vi "AB_Engine_Check_for_nonVI_Link.vi"(1 "buttons":u16, 2 "type":T1) -> (7 "nonVIlink":bool)   [LabVIEW 2020]
uses:
  <vilib>/Utility/lvfile.llb/LVFileType.ctl
  <vilib>/Utility/lvfile.llb/NI_FileType.lvlib
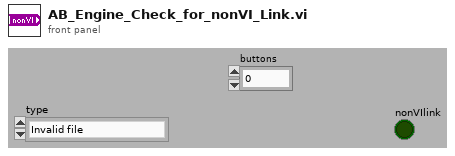
[diagram p1: front panel]
types:
  T1 = typedef "NI_FileType.lvlib/LVFileType.ctl" = enum32{"Invalid file", "Unknown type", "Instrument", "Control", "Polymorphic VI", "Project", "Library", "LVClass", "XControl", "XNode", "Shared library", ".NET assembly", "ActiveX interface", "CIN", "Run-time menu", "Palette menu", "Help file", "LLB", "XNode Edit Dependency", "Class Private Data Control", "Statechart", "MathScript .m file", "Ladder Diagram", "LVLibp", "XNode Build Dependency"}
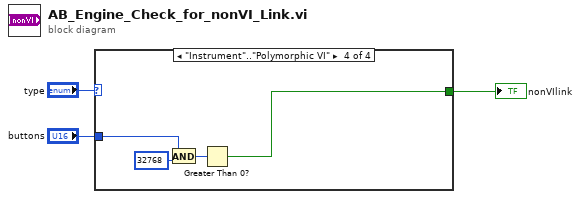
[diagram p0: block diagram]
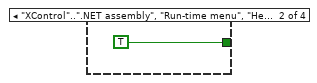
[diagram p3: hidden frame]
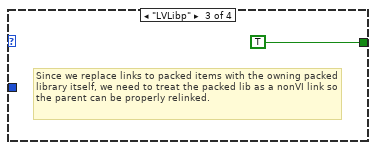
[diagram p4: hidden frame]
diagram:
  n1 = case shown="\"Instrument\"..\"Polymorphic VI\"" "type" {
    tunnel: [_ TRUE TRUE w6] -> w3
    tunnel: "buttons" -> [_ _ _ w7]
    frame Default {
    }
    frame "XControl"..".NET assembly", "Run-time menu", "Help file", "XNode Edit Dependency", "MathScript .m file" {
    }
    frame "LVLibp" {
      # "Since we replace links to packed items with the owning packed library itself, we need to treat the packed lib as a nonVI link so the parent can be properly relinked."
    }
    frame "Instrument".."Polymorphic VI" {
      n2 = And(x=w7, y=u16 32768) -> (x .and. y?=w8:u16)
      n3 = Greater Than 0?(x=w8) -> (x > 0?=w6:bool)
    }
  }
  "nonVIlink" <- w3
